vi "TestCode.vi"() -> ()   [LabVIEW 2012]
uses:
  <userlib>/rosforlv/Gazebo/AxesDrawing/ReferenceFrame.ctl
panel:
  out "sdf out":string
  out "3D Picture":refnum<vi>(3d-picture)
  out "Original Frame":T1={"nx"=1.0, "ny"=0.0, "nz"=0.0, "nw"=0.0, "ox"=0.0, "oy"=0.9999999999999999, "oz"=-1.924386576016938e-17, "ow"=0.0, "ax"=0.0, "ay"=-1.924386576016938e-17, "az"=0.9999999999999999, "aw"=0.0, "Px"=0.0, "Py"=-2.7199999999999998, "Pz"=0.5999999999999996, "Pw"=1.0} {"Pw" format="%.2f"; "Pz" format="%.2f"; "Py" format="%.2f"; "Px" format="%.2f"; "aw" format="%.2f"; "az" format="%.2f"; "ay" format="%.2f"; "ax" format="%.2f"; "ow" format="%.2f"; "nw" format="%.2f"; "oz" format="%.2f"; "oy" format="%.2f"; "ox" format="%.2f"; "nz" format="%.2f"; "ny" format="%.2f"; "nx" format="%.2f"}
  out "Inverse of Final Frame":T1={"nx"=1.0, "ny"=-0.0, "nz"=-0.0, "nw"=-0.0, "ox"=-0.0, "oy"=0.6944444444444444, "oz"=-0.6944444444444444, "ow"=-0.0, "ax"=-0.0, "ay"=0.6944444444444444, "az"=0.6944444444444444, "aw"=-0.0, "Px"=-5.0, "Py"=-3.4722222222222223, "Pz"=-0.6944444444444444, "Pw"=1.0} {"Pw" format="%.2f"; "Pz" format="%.2f"; "Py" format="%.2f"; "Px" format="%.2f"; "aw" format="%.2f"; "az" format="%.2f"; "ay" format="%.2f"; "ax" format="%.2f"; "ow" format="%.2f"; "nw" format="%.2f"; "oz" format="%.2f"; "oy" format="%.2f"; "ox" format="%.2f"; "nz" format="%.2f"; "ny" format="%.2f"; "nx" format="%.2f"}
  out "Final Frame":T1={"nx"=1.0, "ny"=0.0, "nz"=0.0, "nw"=0.0, "ox"=0.0, "oy"=0.72, "oz"=0.72, "ow"=0.0, "ax"=0.0, "ay"=-0.72, "az"=0.72, "aw"=0.0, "Px"=5.0, "Py"=-0.72, "Pz"=3.5999999999999996, "Pw"=1.0} {"Pw" format="%.2f"; "Pz" format="%.2f"; "Py" format="%.2f"; "Px" format="%.2f"; "aw" format="%.2f"; "az" format="%.2f"; "ay" format="%.2f"; "ax" format="%.2f"; "ow" format="%.2f"; "nw" format="%.2f"; "oz" format="%.2f"; "oy" format="%.2f"; "ox" format="%.2f"; "nz" format="%.2f"; "ny" format="%.2f"; "nx" format="%.2f"}
  in  "Rotation 2":T1={"nx"=1.0, "ny"=0.0, "nz"=0.0, "nw"=0.0, "ox"=0.0, "oy"=0.72, "oz"=0.72, "ow"=0.0, "ax"=0.0, "ay"=-0.72, "az"=0.72, "aw"=0.0, "Px"=0.0, "Py"=0.0, "Pz"=0.0, "Pw"=1.0} {"Pw" format="%.2f"; "Pz" format="%.2f"; "Py" format="%.2f"; "Px" format="%.2f"; "aw" format="%.2f"; "az" format="%.2f"; "ay" format="%.2f"; "ax" format="%.2f"; "ow" format="%.2f"; "nw" format="%.2f"; "oz" format="%.2f"; "oy" format="%.2f"; "ox" format="%.2f"; "nz" format="%.2f"; "ny" format="%.2f"; "nx" format="%.2f"}
  in  "Translation 1":T1={"nx"=1.0, "ny"=0.0, "nz"=0.0, "nw"=0.0, "ox"=0.0, "oy"=1.0, "oz"=0.0, "ow"=0.0, "ax"=0.0, "ay"=0.0, "az"=1.0, "aw"=0.0, "Px"=5.0, "Py"=2.0, "Pz"=3.0, "Pw"=1.0} {"Pw" format="%.2f"; "Pz" format="%.2f"; "Py" format="%.2f"; "Px" format="%.2f"; "aw" format="%.2f"; "az" format="%.2f"; "ay" format="%.2f"; "ax" format="%.2f"; "ow" format="%.2f"; "nw" format="%.2f"; "oz" format="%.2f"; "oy" format="%.2f"; "ox" format="%.2f"; "nz" format="%.2f"; "ny" format="%.2f"; "nx" format="%.2f"}
  in  "World Frame":T1={"nx"=1.0, "ny"=0.0, "nz"=0.0, "nw"=0.0, "ox"=0.0, "oy"=1.0, "oz"=0.0, "ow"=0.0, "ax"=0.0, "ay"=0.0, "az"=1.0, "aw"=0.0, "Px"=0.0, "Py"=0.0, "Pz"=0.0, "Pw"=1.0} {"Pw" format="%.2f"; "Pz" format="%.2f"; "Py" format="%.2f"; "Px" format="%.2f"; "aw" format="%.2f"; "az" format="%.2f"; "ay" format="%.2f"; "ax" format="%.2f"; "ow" format="%.2f"; "nw" format="%.2f"; "oz" format="%.2f"; "oy" format="%.2f"; "ox" format="%.2f"; "nz" format="%.2f"; "ny" format="%.2f"; "nx" format="%.2f"}
  # "`"
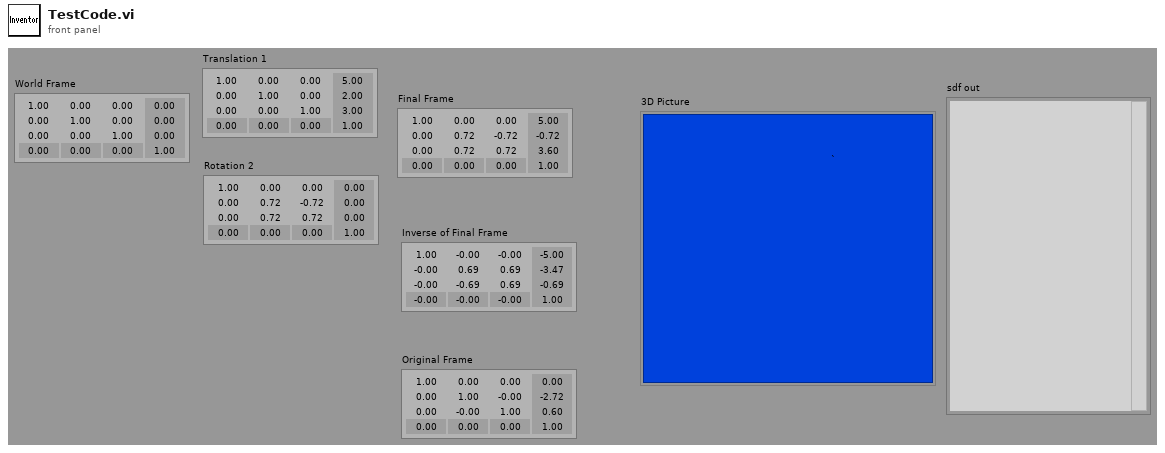
[diagram p1: front panel]
types:
  T1 = typedef "ReferenceFrame.ctl" = cluster{"nx":dbl, "ny":dbl, "nz":dbl, "nw":dbl, "ox":dbl, "oy":dbl, "oz":dbl, "ow":dbl, "ax":dbl, "ay":dbl, "az":dbl, "aw":dbl, "Px":dbl, "Py":dbl, "Pz":dbl, "Pw":dbl}
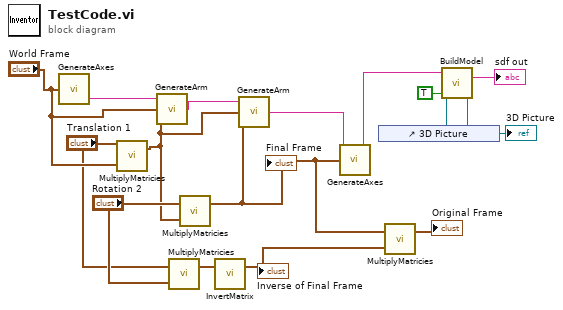
[diagram p0: block diagram]
diagram:
  n1 = call <userlib>:"GenerateAxes.vi"("Frame"="World Frame") -> ("Text Out"=w16:string)  [unwired: 5 in]
  n2 = call <userlib>:"MultiplyMatricies.vi"("B"="World Frame", "A"="Translation 1") -> ("AxB"=w7:T1)  [unwired: 1 out]
  n3 = call <userlib>:"GenerateArm.vi"("Text In"=w16, "Frame Start"="World Frame", "Frame End"=w7) -> ("Text Out"=w2:string)  [unwired: 2 in]
  n4 = call <userlib>:"MultiplyMatricies.vi"("B"="Rotation 2", "A"="Translation 1") -> ("AxB"=w12:T1)  [unwired: 1 out]
  n5 = call <userlib>:"MultiplyMatricies.vi"("B"=w7, "A"="Rotation 2") -> ("AxB"=w11:T1)  [unwired: 1 out]
  "Final Frame" <- w11
  n6 = call <userlib>:"InvertMatrix.vi"("A"=w12) -> ("Inverse of A"=w10:T1)  [unwired: 1 in, 1 out]
  "Inverse of Final Frame" <- w10
  n7 = call <userlib>:"GenerateArm.vi"("Text In"=w2, "Frame Start"=w7, "Frame End"=w11) -> ("Text Out"=w6:string)  [unwired: 2 in]
  n8 = call <userlib>:"GenerateAxes.vi"("Text In"=w6, "Frame"=w11) -> ("Text Out"=w3:string)  [unwired: 4 in]
  n9 = control-ref of="3D Picture"() -> (w1:refnum<vi>)
  n10 = call <userlib>:"MultiplyMatricies.vi"("B"=w10, "A"=w11) -> ("AxB"=→"Original Frame":T1)  [unwired: 1 out]
  n11 = call <userlib>:"BuildModel.vi"(3:TRUE ("Static?"), "3D Picture"=w1, "urdf in"=w3) -> ("3D Picture"=→"3D Picture":refnum<vi>, "urdf out"=→"sdf out":string)  [unwired: 1 in]
